vi "Add Property (String).vi"(7 "Required?":bool, 8 "error in (no error)":errorcluster, 9 "String In":refnum<vi>, 11 "JSON Schema in":string) -> (0 "error out":errorcluster, 3 "JSON SChema out":string)   [LabVIEW 2023, in "JSON Schema Generator.lvlib"]
uses:
  JSON Schema Generator.lvlib
  <vilib>/Utility/Data Type/NI_Data Type.lvlib
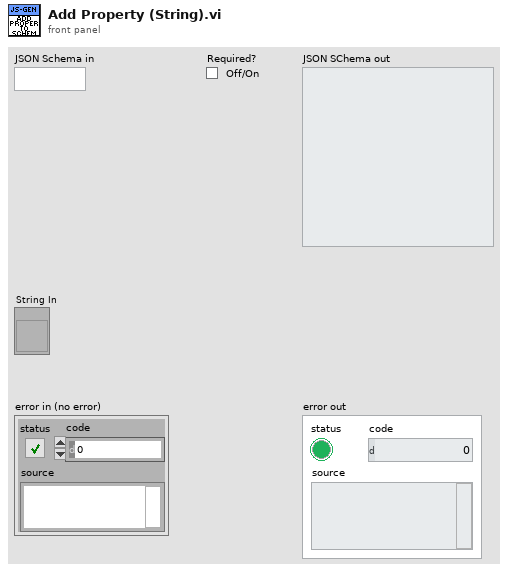
[diagram p1: front panel]
types:
  T1 = typedef "NI_Data Type.lvlib/Data Type.ctl" = enum8{"Invalid Type", "Void", "I8", "I16", "I32", "I64", "U8", "U16", "U32", "U64", "Single Float", "Double Float", "Extended Float", "Single Complex", "Double Complex", "Extended Complex", "Enum U8", "Enum U16", "Enum U32", "Enum U64", "Single Float With Unit", "Double Float With Unit", "Extended Float With Unit", "Single Complex with Unit", "Double Complex with Unit", "Extended Complex with Unit", "Boolean", "String", "Path", "Picture", "Tag", "Array", "Cluster", "Variant", "LV Variant", "Waveform", "Timestamp", "Digital Waveform", "Digital Data", "ExpressData", "Refnum", "External Data", "VI", "Poly VI", "LabVIEW Class Instance", "Fixed Point", "Set Collection", "Map Collection"}
  T2 = typedef "NI_Data Type.lvlib/Type Definition Info.ctl" = cluster{"Name":string, "Timestamp":u32}
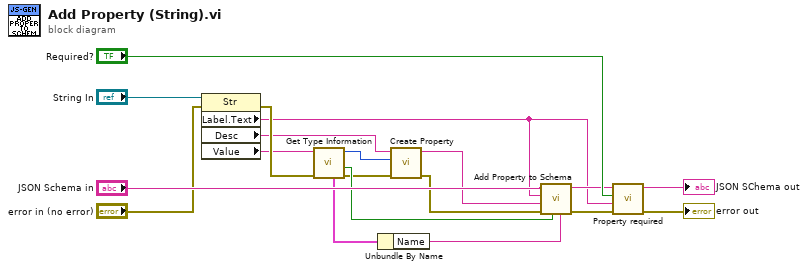
[diagram p0: block diagram]
diagram:
  n1 = property on="Property Node" class="Str"(reference="String In", error in="error in (no error)") -> (error out=w19:errorcluster, "Label.Text"=w7:string, "Desc"=w9:string, "Value"=w10:string)  [unwired: 1 out]
  n2 = call <vilib>:"Get Type Information.vi"("error in (no error)"=w19, "variant"=w10) -> ("error out"=w2:errorcluster, "type definition"=w6:bool, "type"=w8:T1, "type definition info"=w5:T2)  [unwired: 5 in, 1 out]
  n3 = Unbundle By Name(w5) -> ("Name"=w4:string)
  n4 = call "Create Property.vi"("error in"=w2, "Labview Type"=w8, "Description"=w9) -> ("error out"=w1:errorcluster, "JSON Schema Property out"=w13:string)  [unwired: 7 in]
  n5 = call "Add Property to Schema.vi"("Typedef Name"=w4, "Typedef?"=w6, "error in"=w1, "JSON Schema Property in"=w13, "Property Name"=w7, "JSON Schema in"="JSON Schema in") -> ("error out"=w12:errorcluster, "JSON Schema out"=w14:string)  [unwired: 4 in]
  n6 = call "Property required.vi"("error in (no error)"=w12, "Name"=w7, "Required?"="Required?", "JSON Schema in"=w14) -> ("error out"=→"error out":errorcluster, "JSON Schema out"=→"JSON SChema out":string)  [unwired: 6 in]
